vi "Get_exp_data.vi"(8 "error in (no error)":errorcluster, 10 "index":i32, 11 "Control-Client in":refnum<class "Control-Client.lvclass">) -> (0 "error out":errorcluster, 2 "Data":sgl[][](array[numeric]), 3 "Control-Client out":refnum<class "Control-Client.lvclass">)   [LabVIEW 2019, in "Control-Client.lvclass"]
uses:
  Control-Client.lvclass
  Control-Client.lvclass/Control-Client.ctl
  methods/Read Group #.vi
  Experiments/Experiments_group.lvclass
  Experiments/Experiment.lvclass
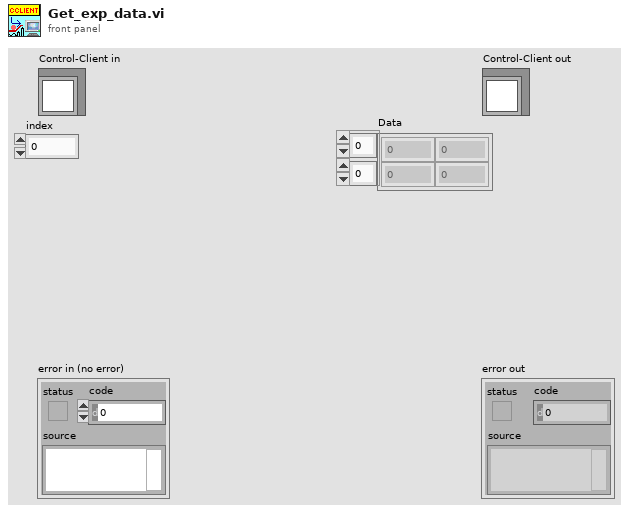
[diagram p1: front panel]
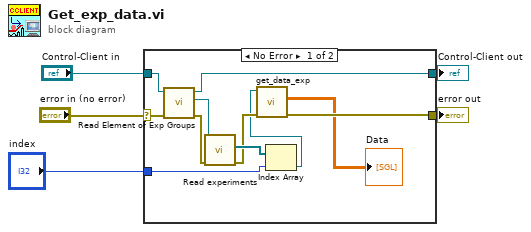
[diagram p0: block diagram]
diagram:
  n1 = case shown="No Error" "error in (no error)" {
    selector: "error in (no error)" -> [w15 w18]
    tunnel: [w9 w18] -> w4
    tunnel: [w14 w17] -> w2
    tunnel: "Control-Client in" -> [w16 w17]
    tunnel: "index" -> [w6 _]
    frame No Error {
      n2 = call "Read Element of Exp Groups.vi"("error in (no error)"=w15, "Control-Client in"=w16) -> ("error out"=w13:errorcluster, "Experiments_group.lvclass"=w12:refnum<class "Experiments_group.lvclass">, "Control-Client out"=w14:refnum<class "Control-Client.lvclass">)  [unwired: 7 in]
      n3 = call "Read experiments.vi"("error in (no error)"=w13, "Experiments_group.lvclass in"=w12) -> ("error out"=w10:errorcluster, "Experiments"=w11:refnum<class "Experiment.lvclass">[])  [unwired: 6 in, 1 out]
      n4 = Index Array(array=w11, index=w6) -> (element=w7:refnum<class "Experiment.lvclass">)
      n5 = call "get_data_exp.vi"("error in (no error)"=w10, "Experiment.lvclass in"=w7) -> ("error out"=w9:errorcluster, "Data"=→"Data":sgl[][])  [unwired: 7 in, 1 out]
    }
    frame Error {
    }
  }
  "error out" <- w4
  "Control-Client out" <- w2
